vi "LVClasse_Phase Set Data.vi"(0 "Phase in":refnum<class "Phase.lvclass">, 5 "data":sgl[][](array[numeric]), 7 "Pupil":refnum<class "Pupil.lvclass">, 11 "error in (no error)":errorcluster) -> (4 "Phase out":refnum<class "Phase.lvclass">, 15 "error out":errorcluster)   [LabVIEW 2020, in "Phase.lvclass"]
doc: "Phase values buffer and pupil setter.\n\n--------------------------------------------------------------------------------\n\n<B>PhaseIn </B> : Phase object.\n<B>PhaseOut </B> : Phase object.\n<B>buffer </B> : Phase values buffer.\n<B>Pupil </B> : pupil object.\n<B>ErrorIn </B> : Error\n<B>ErrorOut </B> : Error\n\n--------------------------------------------------------------------------------"
uses:
  Phase.lvclass
  Pupil/Pupil.lvclass
  Phase.lvclass/Phase.ctl
  Pupil/LVClass_Pupil Read Pupil.vi
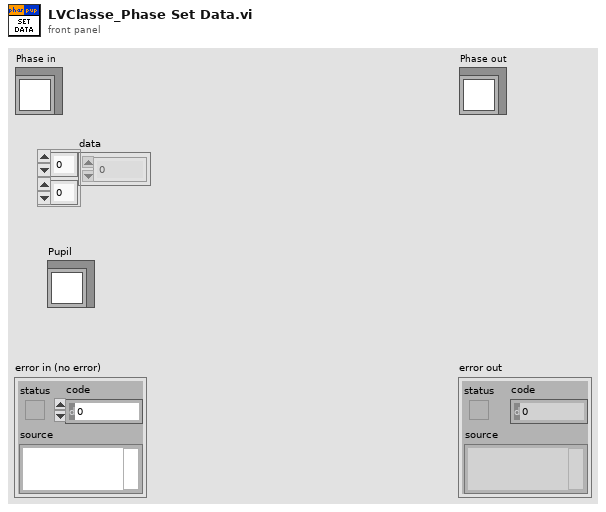
[diagram p1: front panel]
types:
  T1 = typedef "General dimensions definition.ctl" = cluster{"Size":T2, "Step":T3}
  T2 = typedef "Point2D.ctl" = cluster{"X":u32, "Y":u32}
  T3 = typedef "Point2Df.ctl" = cluster{"X":sgl, "Y":sgl}
  T4 = typedef "ClassID.ctl" = i64
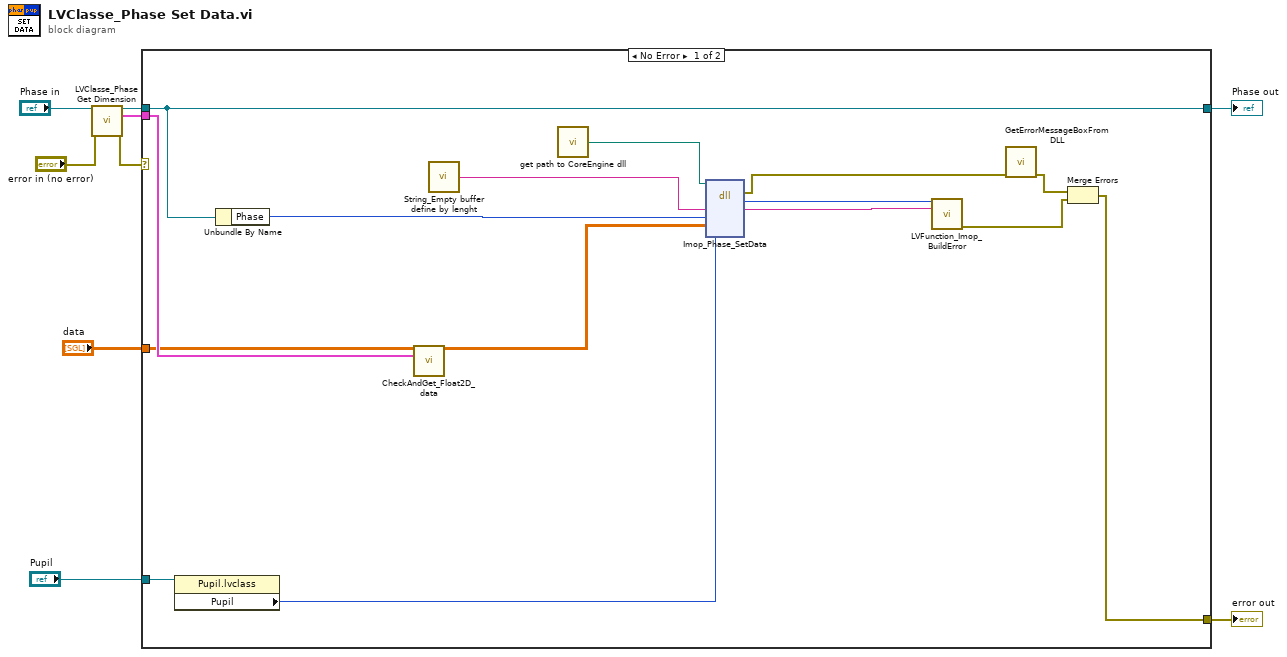
[diagram p0: block diagram]
diagram:
  n1 = call "LVClasse_Phase Get Dimension.vi"("Phase in"="Phase in", "error in (no error)"="error in (no error)") -> ("Phase out"=w5:refnum<class "Phase.lvclass">, "Dimensions_um"=w2:T1, "error out"=w3:errorcluster)  [unwired: 11 in]
  n2 = case shown="No Error" w3 {
    selector: w3 -> [_ w26]
    tunnel: [w13 w26] -> w9
    tunnel: [w19 w25] -> w8
    tunnel: w5 -> [w19 w25]
    tunnel: "Pupil" -> [w17 _]
    tunnel: w2 -> [w12 _]
    tunnel: "data" -> [w11 _]
    frame No Error {
      n3 = property class="Pupil.lvclass"(reference=w17) -> ("Pupil"=w16:T4)  [unwired: 1 in, 2 out]
      n4 = Unbundle By Name(w19) -> ("Phase"=w18:T4)
      n5 = call "CheckAndGet_Float2D_data.vi"("data in"=w11, "Dimensions_um"=w12) -> ("data out"=w10:sgl[][])  [unwired: 13 in]
      n6 = call "String_Empty buffer define by lenght.vi"() -> ("Empty buffer"=w22:string)  [unwired: 1 in]
      n7 = call "get path to CoreEngine dll.vi"() -> ("path to wavekit library"=w21:path)  [unwired: 14 in, 1 out]
      n8 = dll-call lib="D:/2_trunk/Soft_haso/ImOpCoreEngine4_LV2011/DLLs/ImopEngine4_vc100.dll" fn="Imop_Phase_SetData"(path in=w21, "message"=w22, "phase"=w18, "data"=w10, "pupil"=w16) -> (error out=w20:errorcluster, "return type"=w24:i32, "message"=w23:string)  [unwired: 5 in, 1 out]
      n9 = call "LVFunction_Imop_BuildError.vi"("code"=w24, "String to Prepend to source (\"\")"=w23) -> ("error out"=w14:errorcluster)  [unwired: 13 in]
      n10 = call "GetErrorMessageBoxFromDLL.vi"("error IN"=w20) -> ("error OUT"=w15:errorcluster)  [unwired: 10 in]
      n11 = Merge Errors(w15, w14) -> (w13:errorcluster)
    }
    frame Error {
    }
  }
  "error out" <- w9
  "Phase out" <- w8
